vi "Load PlotConfig.vi"(8 "error in (no error)":errorcluster, 9 "Load options (All)":T1={"Load plots?"=TRUE, "Load X-axis?"=TRUE, "Load Y-axes?"=TRUE, "Load General?"=TRUE}, 10 "Plot config":T2={"plots"=[], "X-axis"={"Name Label.Text"="", "Style"=0, "Tick Colors:Minor Tick Color"=0, "Tick Colors:Tick Color"=0, "Marker Colors:Text Color"=0, "Grid Colors:Major Color"=0, "Grid Colors:Minor Color"=0, "Mapping Mode"=0, "Flipped"=FALSE, "Name Label.Visible"=FALSE, "Name Label.Text Colors:Text Color"=0, "Scale Fit"=0, "Range:Maximum"=0.0, "Range:Minimum"=0.0, "Offset and Multiplier:Multiplier"=0.0, "Offset and Multiplier:Offset"=0.0, "Name Label.Font:Size"=0, "Marker.Font:Size"=0, "Uniform Marker Spacing?"=TRUE, "Format String"=""}, "Y-axes"=[], "General"={"Title"="", "Time to Plot"=1800.0, "Title.Visible"=FALSE, "Sidebar.Visible"=FALSE, "Plot Area:Colors:BG Color"=0, "X Scale.Plot Name"="", "X Scale.Use Plot Name"=FALSE}} {"General"."Time to Plot" format="%<%M:%S>t"}, 11 "BluePlotHandle in":refnum<class "RocketPlotHandle.lvclass">) -> (0 "error out":errorcluster, 3 "BluePlotHandle out":refnum<class "RocketPlotHandle.lvclass">)   [LabVIEW 2021, in "RocketPlotHandle.lvclass"]
doc: "Load plot configuration into the attached plot instance.\n\nNote that this will load ALL plot settings from the input \"plot config\" cluster input.\nThere is no mechanism for specifying only a subset of these settings to be loaded.\nIt's all or nothin'\n\nIf you ever needed to modify/load only 1 aspect of a plot, then I recommend:\n- perform \"get plot config\"\n- perform in-place modification of the plot config cluster to adjust what you want to specifically change\n- perform \"load plot config\""
uses:
  RocketPlotHandle.lvclass
  TypeDefs/plot load data V2.ctl
  TypeDefs/plot properties V2.ctl
  TypeDefs/plot attributes V2.ctl
  TypeDefs/Plot scale axis properties.ctl
  TypeDefs/Plot general properties.ctl
  SubVIs/Load config options.ctl
  RocketPlotHandle.lvclass/RocketPlotHandle.ctl
  TypeDefs/plot handle queue data.ctl
  TypeDefs/Plot QSM action.ctl
  SubVIs/Load config.ctl
  RocketPlot.lvlib
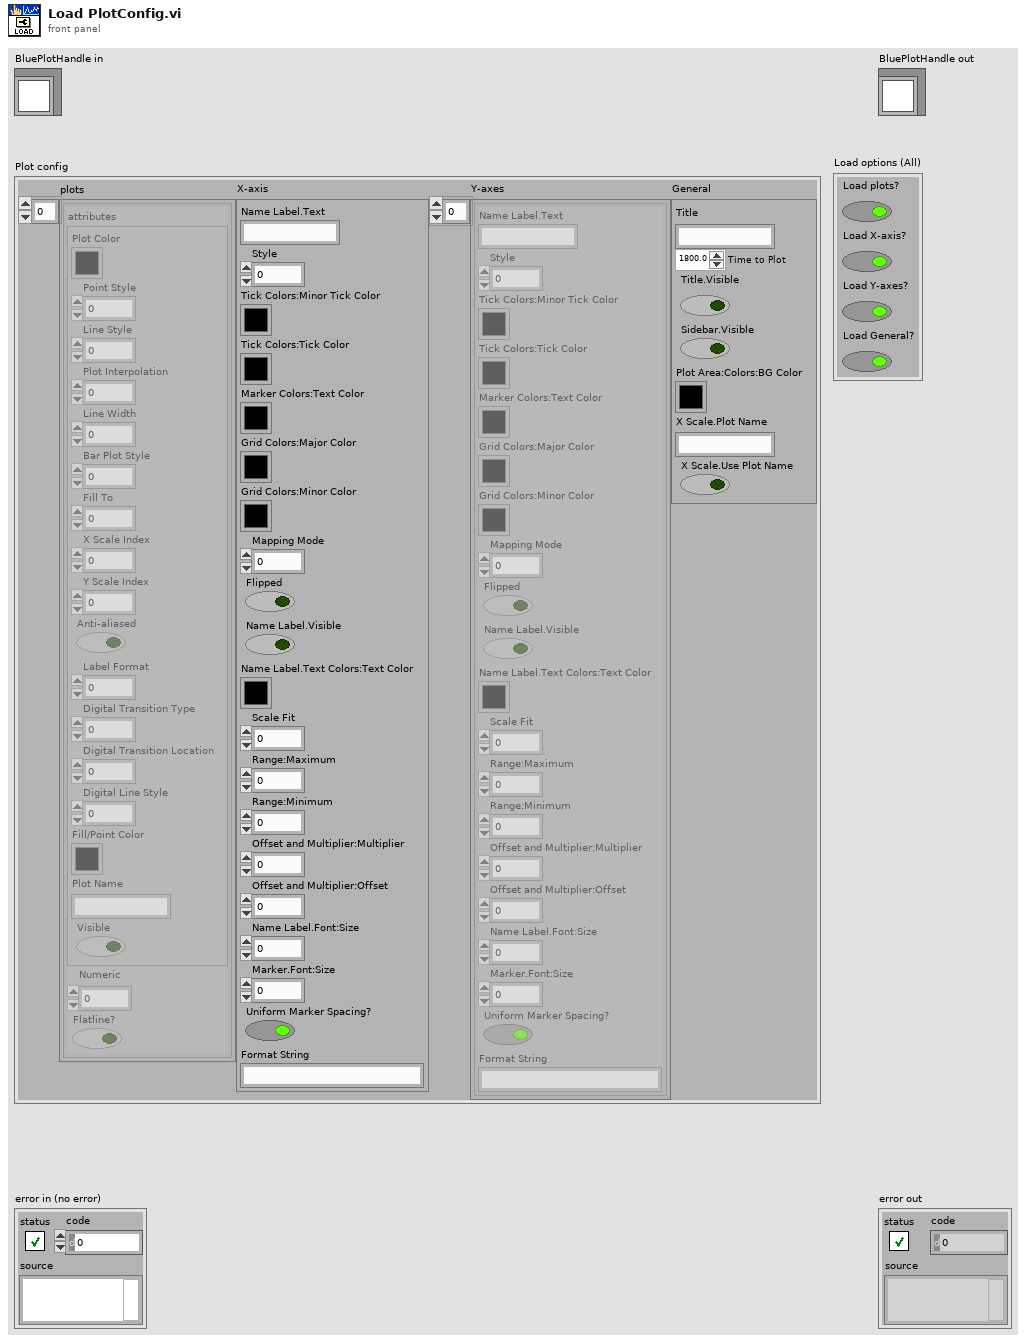
[diagram p1: front panel]
types:
  T1 = typedef "RocketPlotHandle.lvclass/Load config options.ctl" = cluster{"Load plots?":bool, "Load X-axis?":bool, "Load Y-axes?":bool, "Load General?":bool}
  T2 = typedef "RocketPlot.lvlib/plot load data V2.ctl" = cluster{"plots":T3[], "X-axis":T5, "Y-axes":T5[], "General":T6}
  T3 = typedef "RocketPlot.lvlib/plot properties V2.ctl" = cluster{"attributes":T4, "Numeric":dbl, "Flatline?":bool}
  T4 = typedef "RocketPlot.lvlib/plot attributes V2.ctl" = cluster{"Plot Color":u32, "Point Style":u8, "Line Style":u8, "Plot Interpolation":u8, "Line Width":u8, "Bar Plot Style":u8, "Fill To":i16, "X Scale Index":u32, "Y Scale Index":u32, "Anti-aliased":bool, "Label Format":u8, "Digital Transition Type":u8, "Digital Transition Location":u8, "Digital Line Style":u8, "Fill/Point Color":u32, "Plot Name":string, "Visible":bool}
  T5 = typedef "RocketPlot.lvlib/Plot scale axis properties.ctl" = cluster{"Name Label.Text":string, "Style":u8, "Tick Colors:Minor Tick Color":u32, "Tick Colors:Tick Color":u32, "Marker Colors:Text Color":u32, "Grid Colors:Major Color":u32, "Grid Colors:Minor Color":u32, "Mapping Mode":u8, "Flipped":bool, "Name Label.Visible":bool, "Name Label.Text Colors:Text Color":u32, "Scale Fit":u8, "Range:Maximum":dbl, "Range:Minimum":dbl, "Offset and Multiplier:Multiplier":dbl, "Offset and Multiplier:Offset":dbl, "Name Label.Font:Size":u32, "Marker.Font:Size":u32, "Uniform Marker Spacing?":bool, "Format String":string}
  T6 = typedef "RocketPlot.lvlib/Plot general properties.ctl" = cluster{"Title":string, "Time to Plot":dbl, "Title.Visible":bool, "Sidebar.Visible":bool, "Plot Area:Colors:BG Color":u32, "X Scale.Plot Name":string, "X Scale.Use Plot Name":bool}
  T7 = typedef "RocketPlotHandle.lvclass/Load config.ctl" = cluster{"Plot config":T2, "Load options (All)":T1}
  T8 = typedef "RocketPlot.lvlib/Plot QSM action.ctl" = enum16{"Get Config", "Load Config", "Set TimeToPlot", "Clear Config"}
  T9 = typedef "RocketPlot.lvlib/plot handle queue data.ctl" = cluster{"action":T8, "data":variant}
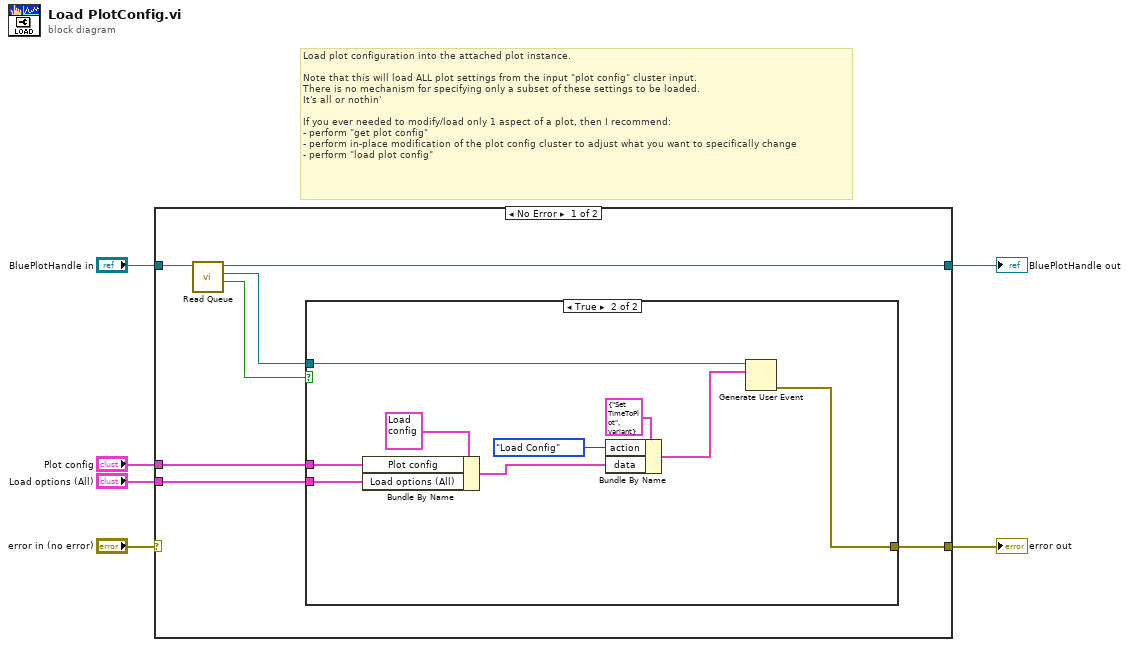
[diagram p0: block diagram]
diagram:
  # "Load plot configuration into the attached plot instance.\n\nNote that this will load ALL plot settings from the input \"plot config\" cluster input.\nThere is no mechanism for specifying only a subset of these settings to be loaded.\nIt's all or nothin'\n\nIf you ever needed to modify/load only 1 aspect of a plot, then I recommend:\n- perform \"get plot config\"\n- perform in-place modification of the plot config cluster to adjust what you want to specifically change\n- perform \"load plot config\""
  n1 = case shown="No Error" "error in (no error)" {
    selector: "error in (no error)" -> [_ w24]
    tunnel: "BluePlotHandle in" -> [w12 w23]
    tunnel: [w9 w24] -> w5
    tunnel: [w10 w23] -> w3
    tunnel: "Plot config" -> [w8 _]
    tunnel: "Load options (All)" -> [w7 _]
    frame No Error {
      n2 = call "Read Queue.vi"("BluePlotHandle in"=w12) -> ("Valid?"=w13:bool, "UE"=w11:refnum<user-event>, "BluePlotHandle out"=w10:refnum<class "RocketPlotHandle.lvclass">)  [unwired: 8 in]
      n3 = case shown="True" w13 {
        tunnel: w11 -> [_ w22]
        tunnel: [_ w18] -> w9
        tunnel: w8 -> [_ w16]
        tunnel: w7 -> [_ w15]
        frame False {
        }
        frame True {
          n4 = Bundle By Name(cluster=T7 {"Plot config"={"plots"=[], "X-axis"={"Name Label.Text"="", "Style"=0, "Tick Colors:Minor Tick Color"=0, "Tick Colors:Tick Color"=0, "Marker Colors:Text Color"=0, "Grid Colors:Major Color"=0, "Grid Colors:Minor Color"=0, "Mapping Mode"=0, "Flipped"=FALSE, "Name Label.Visible"=FALSE, "Name Label.Text Colors:Text Color"=0, "Scale Fit"=0, "Range:Maximum"=0.0, "Range:Minimum"=0.0, "Offset and Multiplier:Multiplier"=0.0, "Offset and Multiplier:Offset"=0.0, "Name Label.Font:Size"=0, "Marker.Font:Size"=0, "Uniform Marker Spacing?"=TRUE, "Format String"=""}, "Y-axes"=[], "General"={"Title"="", "Time to Plot"=1800.0, "Title.Visible"=FALSE, "Sidebar.Visible"=FALSE, "Plot Area:Colors:BG Color"=0, "X Scale.Plot Name"="", "X Scale.Use Plot Name"=FALSE}}, "Load options (All)"={"Load plots?"=TRUE, "Load X-axis?"=TRUE, "Load Y-axes?"=TRUE, "Load General?"=TRUE}} ("Cluster"), "Plot config"=w16, "Load options (All)"=w15) -> (w14:T7)
          n5 = Bundle By Name(cluster=T9 {"action"=enum."Set TimeToPlot", "data"=variant} ("element"), "action"=Plot_QSM_action."Load Config", "data"=w14) -> (w19:T9)
          n6 = Generate User Event(user event=w22, event data cluster=w19) -> (error out=w18:errorcluster)  [unwired: 2 in, 1 out]
        }
      }
    }
    frame Error {
    }
  }
  "BluePlotHandle out" <- w3
  "error out" <- w5
